vi "ADCP_Get_Packet_Info_From_Processed_Packet.vi"(8 "error in (no error)":errorcluster, 10 "Processed Packet":u8[](array[numeric])=[0, 0, 0, 0, 0, 0, 0, 0, 0], 11 "ADCP in":refnum<class "ADCP.lvclass">) -> (0 "error out":errorcluster, 2 "Checksum Valid ?":bool, 3 "ADCP out":refnum<class "ADCP.lvclass">, 4 "Packet frame ID":u8, 5 "Packet Type":T1(ring), 6 "Packet node ID":u8, 7 "Packet_Priority":enum16{"LOW", "HIGH"}(ring))   [LabVIEW 2017, in "ADCP.lvclass"]
uses:
  ADCP.lvclass
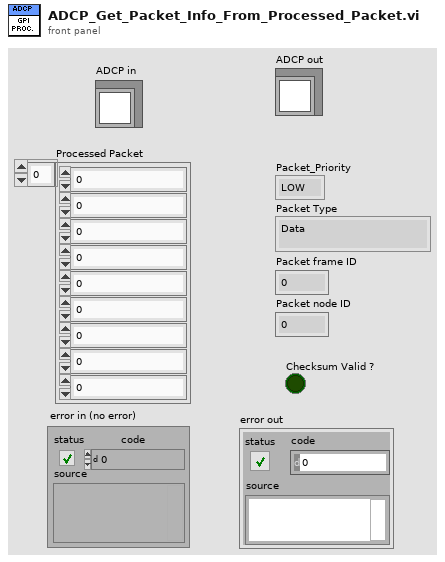
[diagram p1: front panel]
types:
  T1 = enum16{"Data", "Connection Management", "Remote Request", "Error and status", "INVALID"}
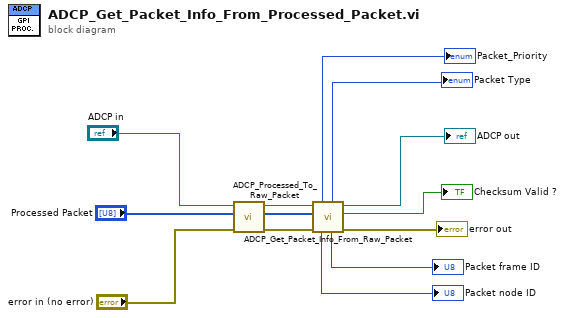
[diagram p0: block diagram]
diagram:
  n1 = call "ADCP_Processed_To_Raw_Packet.vi"("error in (no error)"="error in (no error)", "Processed Packet"="Processed Packet", "ADCP in"="ADCP in") -> ("error out"=w10:errorcluster, "Raw Packet"=w9:u8[], "ADCP out"=w8:refnum<class "ADCP.lvclass">)  [unwired: 6 in]
  n2 = call "ADCP_Get_Packet_Info_From_Raw_Packet.vi"("error in (no error)"=w10, "Raw Packet"=w9, "ADCP in"=w8) -> ("error out"=→"error out":errorcluster, "Checksum Valid ?"=→"Checksum Valid ?":bool, "ADCP out"=→"ADCP out":refnum<class "ADCP.lvclass">, "Packet frame ID"=→"Packet frame ID":u8, "Packet Type"=→"Packet Type":T1, "Packet node ID"=→"Packet node ID":u8, "Packet_Priority"=→"Packet_Priority":enum16{"LOW", "HIGH"})  [unwired: 2 in]
